vi "Draw Flat Top Filled Triangle.vi"(4 "Fill Colour":u32(colorbox), 8 "Point 3":T1, 9 "Point 2":T1, 10 "Point 1":T1, 11 "Pixel Data in":u32[][](array[numeric])) -> (3 "Pixel Data out":u32[][](array[numeric]))   [LabVIEW 2020, in "Raster.lvlib"]
uses:
  Raster.lvlib
  Point 2D.ctl
  Utility/Delta Time.vi
  <vilib>/Utility/High Resolution Relative Seconds.vi
panel:
  out "x+y":i32
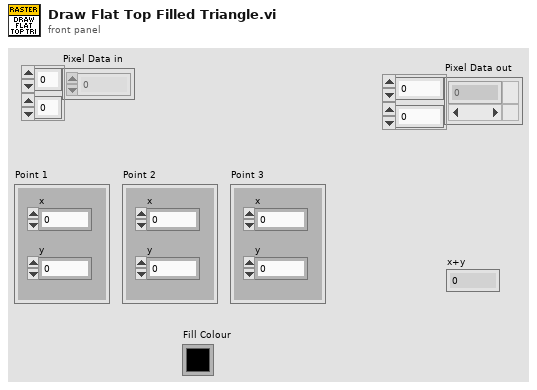
[diagram p1: front panel]
types:
  T1 = typedef "Raster.lvlib/Point 2D.ctl" = cluster{"x":i32, "y":i32}
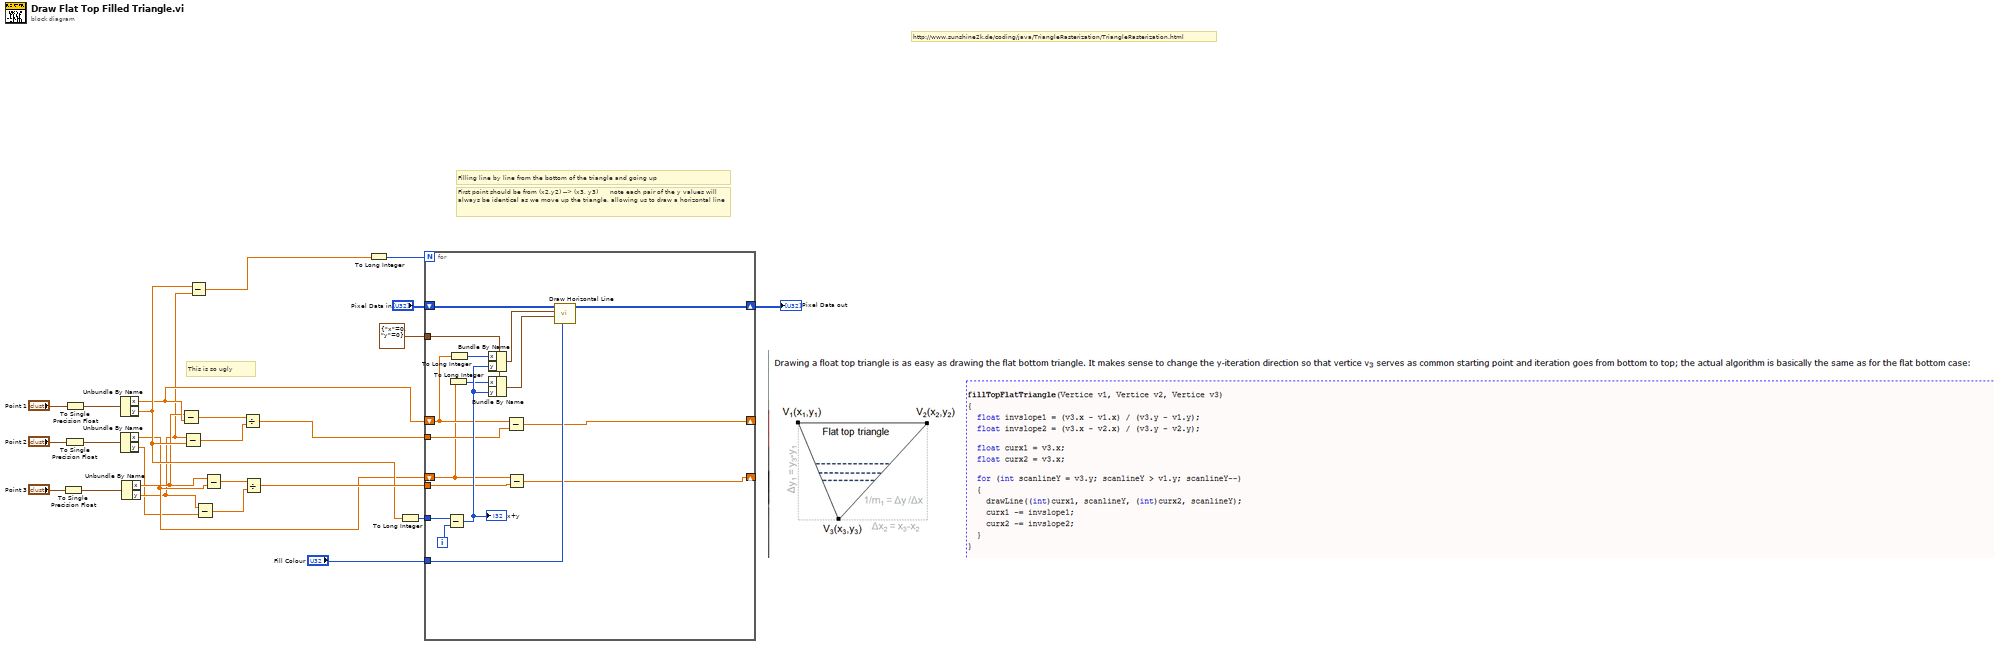
[diagram p0: block diagram]
diagram:
  # "This is so ugly"
  # "First point should be from (x2,y2) --> (x3, y3)      note each pair of the y values will always be identical as we move up the triangle, allowing us to draw a horizontal line"
  # "Filling line by line from the bottom of the triangle and going up"
  # "http://www.sunshine2k.de/coding/java/TriangleRasterization/TriangleRasterization.html"
  n1 = To Single Precision Float(number="Point 3") -> (single precision float=w17:cluster{"x":sgl, "y":sgl})
  n2 = To Single Precision Float(number="Point 2") -> (single precision float=w19:cluster{"x":sgl, "y":sgl})
  n3 = To Single Precision Float(number="Point 1") -> (single precision float=w21:cluster{"x":sgl, "y":sgl})
  n4 = Unbundle By Name(w21) -> ("x"=w6:sgl, "y"=w7:sgl)
  n5 = Unbundle By Name(w19) -> ("x"=w4:sgl, "y"=w2:sgl)
  n6 = Unbundle By Name(w17) -> ("x"=w5:sgl, "y"=w3:sgl)
  n7 = Subtract(x=w5, y=w6) -> (x-y=w24:sgl)
  n8 = Subtract(x=w3, y=w7) -> (x-y=w15:sgl)
  n9 = Subtract(x=w7, y=w3) -> (x-y=w9:sgl)
  n10 = Subtract(x=w3, y=w2) -> (x-y=w16:sgl)
  n11 = Subtract(x=w5, y=w4) -> (x-y=w23:sgl)
  n12 = Divide(x=w24, y=w15) -> (x/y=w11:sgl)
  n13 = Divide(x=w23, y=w16) -> (x/y=w10:sgl)
  n14 = To Long Integer(number=w9) -> (32bit integer=w8:i32)
  n15 = To Long Integer(number=w7) -> (32bit integer=w12:i32)
  n16 = for {
    N: w8 -> [_]
    shift-right: [w27] -> w1
    shift-left: "Pixel Data in" -> [w42]
    tunnel: T1 {"x"=0, "y"=0} ("Point 1") -> [w41]
    tunnel: "Fill Colour" -> [w38]
    shift-right: [w30] -> _
    shift-left: w6 -> [w33]
    shift-right: [w31] -> _
    shift-left: w4 -> [w28]
    tunnel: w12 -> [w35]
    tunnel: w11 -> [w32]
    tunnel: w10 -> [w29]
    i -> [w26]
    n17 = Subtract(x=w35, y=w26) -> (x-y=w36:i32)
    "x+y" <- w36
    n18 = To Long Integer(number=w28) -> (32bit integer=w34:i32)
    n19 = To Long Integer(number=w33) -> (32bit integer=w37:i32)
    n20 = Bundle By Name(cluster=w41, "x"=w37, "y"=w36) -> (w40:T1)
    n21 = Bundle By Name(cluster=w41, "x"=w34, "y"=w36) -> (w39:T1)
    n22 = Subtract(x=w33, y=w32) -> (x-y=w30:sgl)
    n23 = Subtract(x=w28, y=w29) -> (x-y=w31:sgl)
    n24 = call "Draw Horizontal Line.vi"("Colour"=w38, "Point 2"=w39, "Point 1"=w40, "Pixel Data in"=w42) -> ("Pixel Data out"=w27:u32[][])  [unwired: 7 in]
  }
  "Pixel Data out" <- w1
